vi "WriteClusterSettings.vi"(0 "reference in":refnum<class "Logger.lvclass">, 5 "Event":T1={"obj_tag"="", "event_tag"="", "code"=enum."DI_RAW_LO", "Priority"=enum."Alert", "Value"=0.0, "Description"="", "Time Stamp"=timestamp(0 s since 1904-01-01)}, 11 "error in (no error)":errorcluster) -> (4 "reference out":refnum<class "Logger.lvclass">, 15 "error out":errorcluster)   [LabVIEW 2019, in "Logger.lvclass"]
uses:
  Logger.lvclass
  EventData.ctl
  EventCode.ctl
  Priority.ctl
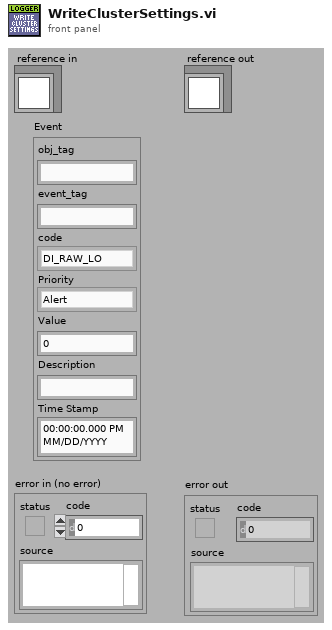
[diagram p1: front panel]
types:
  T1 = typedef "Logger.lvclass/EventData.ctl" = cluster{"obj_tag":string, "event_tag":string, "code":T2, "Priority":T3, "Value":dbl, "Description":string, "Time Stamp":timestamp}
  T2 = typedef "Logger.lvclass/EventCode.ctl" = enum16{"DI_EU_LO", "DI_EU_HI", "DIO_LO", "DIO_HI", "DI_RAW_LO", "DI_RAW_HI", "DO_LO", "DO_HI", "DA_OK", "DA_ALARM", "AA_HI", "AA_HIHI", "AA_LO", "AA_LOLO", "AA_OK", "CMD", "OUT_OF_RANGE_OK", "OUT_OF_RANGE_LO", "OUT_OF_RANGE_HI"}
  T3 = typedef "Logger.lvclass/Priority.ctl" = enum16{"Alert", "Critical", "Error", "Warning", "Notice", "Informational", "Debug"}
  T4 = typedef "Logger.lvclass/ObjectAttributes.ctl" = cluster{"queue_event":refnum<queue>, "DatabaseInterface":refnum<class "DatabaseInterface.lvclass">, "queue_device":refnum<queue>, "queue_signals":refnum<queue>}
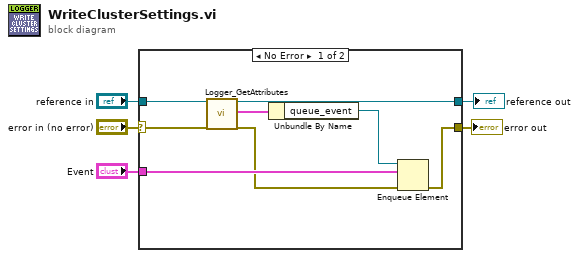
[diagram p0: block diagram]
diagram:
  n1 = case shown="No Error" "error in (no error)" {
    selector: "error in (no error)" -> [w13 w15]
    tunnel: [w7 w15] -> w4
    tunnel: [w12 w14] -> w2
    tunnel: "reference in" -> [w10 w14]
    tunnel: "Event" -> [w8 _]
    frame No Error {
      n2 = call "Logger_GetAttributes.vi"("reference in"=w10, "error in (no error)"=w13) -> ("reference out"=w12:refnum<class "Logger.lvclass">, "attributes"=w11:T4, "error out"=w6:errorcluster)  [unwired: 14 in, 1 out]
      n3 = Unbundle By Name(w11) -> ("queue_event"=w9:refnum<queue>)
      n4 = Enqueue Element(queue=w9, element=w8, error in (no error)=w6) -> (error out=w7:errorcluster)  [unwired: 1 in, 2 out]
    }
    frame Error {
    }
  }
  "error out" <- w4
  "reference out" <- w2
